vi "resultsColumnsTravOffset.vi"(10 "chValuesIn":string[](array[string]), 11 "chNamesIn":string[](array[string])) -> (2 "chValuesOut":string[](array[string]), 3 "chNamesOut":string[](array[string]))   [LabVIEW 2020]
uses:
  Globals/Trav_pos_global.vi
  Globals/Meas_global.vi
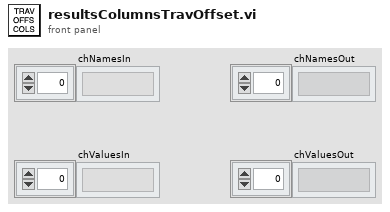
[diagram p1: front panel]
types:
  T1 = typedef "Post_Process.ctl" = enum16{"Take New Data", "Post Process Raw Data File"}
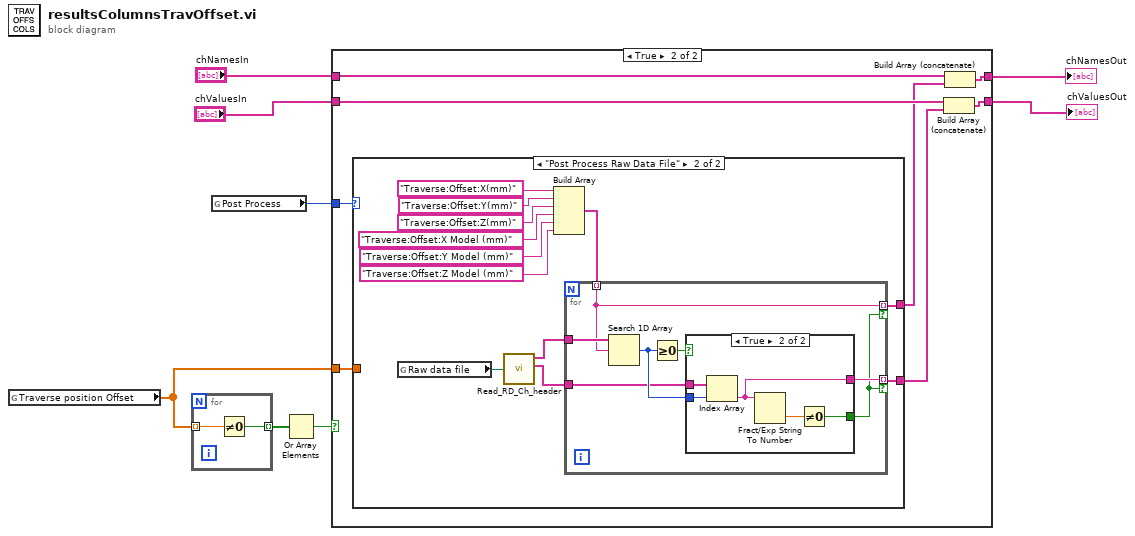
[diagram p0: block diagram]
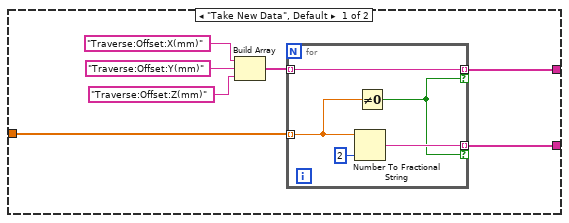
[diagram p3: hidden frame]
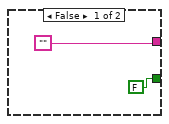
[diagram p4: hidden frame]
diagram:
  n1 = global read "Trav_pos_global.vi" "Traverse position Offset"() -> (w7:sgl[])
  n2 = for {
    tunnel: w7 -> [w10] mode=indexing
    tunnel: [w9] -> w6 mode=indexing
    n3 = Not Equal To 0?(x=w10) -> (x != 0?=w9:bool)
  }
  n4 = global read "Meas_global.vi" "Post Process"() -> (w1:T1)
  n5 = Or Array Elements(Boolean array=w6) -> (logical OR=w8:bool)
  n6 = case shown="True" w8 {
    tunnel: "chValuesIn" -> [w11 w19]
    tunnel: "chNamesIn" -> [w12 w18]
    tunnel: [w12 w16] -> w4
    tunnel: [w11 w15] -> w5
    tunnel: w7 -> [_ w14]
    tunnel: w1 -> [_ w13]
    frame False {
    }
    frame True {
      n7 = case shown="\"Post Process Raw Data File\"" w13 {
        tunnel: [w27 w34] -> w20
        tunnel: [w23 w35] -> w17
        tunnel: w14 -> [w21 _]
        frame "Take New Data", Default {
          n8 = Build Array("Traverse:Offset:X(mm)", "Traverse:Offset:Y(mm)", "Traverse:Offset:Z(mm)") -> (w22:string[])
          n9 = for {
            tunnel: [w32] -> w27 mode=indexing if=w28
            tunnel: w21 -> [w30] mode=indexing
            tunnel: [w29] -> w23 mode=indexing if=w28
            tunnel: w22 -> [w29] mode=indexing
            n10 = Number To Fractional String(number=w30, precision (6)=i16 2) -> (F-format string=w32:string)  [unwired: 2 out]
            n11 = Not Equal To 0?(x=w30) -> (x != 0?=w28:bool)
          }
        }
        frame "Post Process Raw Data File" {
          n12 = global read "Meas_global.vi" "Raw data file"() -> (w33:path)
          n13 = call "Read_RD_Ch_header.vi"("Raw data file"=w33) -> ("Ch Name Out"=w41:string[], "Ch Values"=w40:string[])  [unwired: 2 out]
          n14 = Build Array("Traverse:Offset:X(mm)", "Traverse:Offset:Y(mm)", "Traverse:Offset:Z(mm)", "Traverse:Offset:X Model (mm)", "Traverse:Offset:Y Model (mm)", "Traverse:Offset:Z Model (mm)") -> (w36:string[])
          n15 = for {
            tunnel: w41 -> [w51]
            tunnel: w40 -> [w48]
            tunnel: w36 -> [w46] mode=indexing
            tunnel: [w47] -> w34 mode=indexing if=w45
            tunnel: [w46] -> w35 mode=indexing if=w45
            n16 = Search 1D Array(1D array=w51, element=w46) -> (index of element=w49:i32)  [unwired: 1 out]
            n17 = Greater Or Equal To 0?(x=w49) -> (x >= 0?=w50:bool)
            n18 = case shown="True" w50 {
              tunnel: w49 -> [_ w58]
              tunnel: w48 -> [_ w57]
              tunnel: ["" w55] -> w47
              tunnel: [FALSE w54] -> w45
              frame False {
              }
              frame True {
                n19 = Index Array(array=w57, index=w58) -> (element=w55:string)
                n20 = Fract/Exp String To Number(string=w55) -> (number=w56:dbl)  [unwired: 3 in, 1 out]
                n21 = Not Equal To 0?(x=w56) -> (x != 0?=w54:bool)
              }
            }
          }
        }
      }
      n22 = Build Array (concatenate)(w19, w20) -> (w15:string[])
      n23 = Build Array (concatenate)(w18, w17) -> (w16:string[])
    }
  }
  "chValuesOut" <- w5
  "chNamesOut" <- w4
